vi "Begin.vi"(8 "error in":errorcluster) -> (0 "error out":errorcluster)   [LabVIEW 2016]
doc: "Called before other user functions, this VI is expected to open initial I/O refnums, load in file data, and do all program initialization. Notice that the <B>error out</B> terminal is simply used for data flow. Wiring it to other structures or subVIs ensures that this VI runs first."
uses:
  <vilib>/Rock Robotics/WPI/Camera/WPI_CameraImageSize.ctl
  <vilib>/Rock Robotics/WPI/DriverStation/WPI_DriverStationRobotMode2.ctl
  <vilib>/Rock Robotics/WPI/Joystick/WPI_JoystickDeviceEnum.ctl
  <vilib>/Rock Robotics/WPI/ThirdParty/CanMotor/TalonSRX/WPI_CANTalonSRX_BrakeOverride.ctl
  <vilib>/Rock Robotics/WPI/Solenoid/WPI_SolenoidChannel.ctl
  <vilib>/Rock Robotics/SystemInterfaces/DIO/FPGA_DIOChannel.ctl
  <vilib>/Rock Robotics/SystemInterfaces/DIO/FPGA_DIOPWMChannel.ctl
  <vilib>/Rock Robotics/WPI/ThirdParty/CanMotor/TalonSRX/WPI_CANTalonSRX_StatusFrame.ctl
  <vilib>/Rock Robotics/SystemInterfaces/AI/FPGA_AIChannel.ctl
  <vilib>/Rock Robotics/SystemInterfaces/DIO/FPGA_DIORelayChannel.ctl
  <vilib>/Rock Robotics/SystemInterfaces/spilib/spi_bus.ctl
  Robot Global Data.vi
  <vilib>/Rock Robotics/WPI/Utilities/WPI_GetSetVariantRefNum.vi
  <vilib>/Rock Robotics/WPI/Solenoid/WPI_SolenoidOpenSingle.vi
  <vilib>/Rock Robotics/WPI/MotorControl/WPI_MotorControlOpen VictorSP.vi
  <vilib>/Rock Robotics/WPI/Counter/WPI_CounterDigitalInputToDigitalSource.vi
  navX.Library.v2/navX Library v2/IO/Open/Z900_navX_Open_SPI.vi
  <vilib>/Rock Robotics/WPI/ThirdParty/CanMotor/TalonSRX/WPI_CANTalonSRX_APIControlMode.ctl
  <vilib>/Rock Robotics/WPI/Camera/WPI_CameraWhite Balance Values.ctl
  <vilib>/Rock Robotics/WPI/Camera/WPI_CameraExposure Values.ctl
  <vilib>/Rock Robotics/WPI/Ultrasonic/WPI_SonarSRF04DigitalOpen.vi
  <vilib>/Rock Robotics/WPI/Ultrasonic/WPI_SonarSRF04DigitalRefNum Registry Set.vi
  navX-MXP Library/navX-MXP IMU.lvlib
  navX-MXP Library/COMMON/TypeDefs/Value TypeDefs/navX Interface Protocol.ctl
  navX-MXP Library/COMMON/TypeDefs/Value TypeDefs/navX Update Rate.ctl
  <vilib>/Rock Robotics/WPI/AnalogOutput/WPI_AnalogOutputChannel.ctl
  <vilib>/Rock Robotics/WPI/Camera/WPI_CameraFrameRate.ctl
  navX.Library.v2/navX Library v2/navX Library v2.lvlib
  <vilib>/Rock Robotics/WPI/MotorControl/WPI_MotorControlOpen SD540.vi
panel:
  in  "Image Size":T1=enum."320x240"
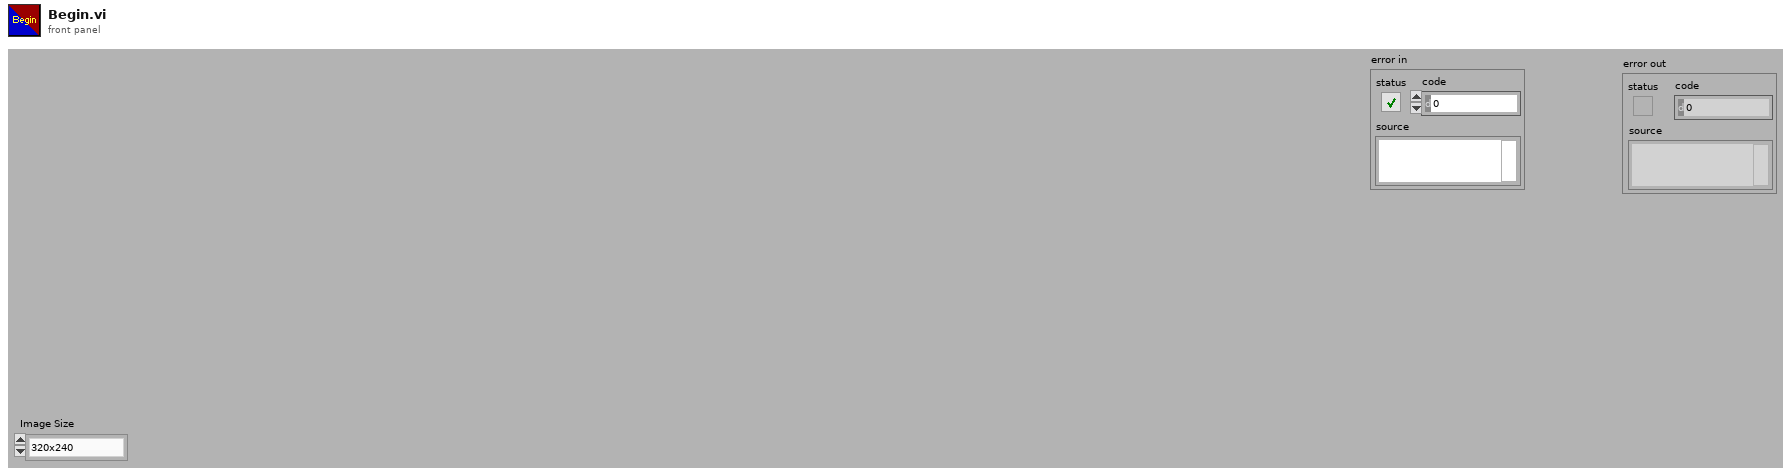
[diagram p1: front panel]
types:
  T1 = typedef "WPI_CameraImageSize.ctl" = enum16{"640x480", "320x240", "160x120", "Custom"}
  T2 = typedef "FPGA_DIORelayChannel.ctl" = enum8{"Relay 0", "Relay 1", "Relay 2", "Relay 3", "Invalid"}
  T3 = typedef "FPGA_DIOPWMChannel.ctl" = enum8{"PWM 0", "PWM 1", "PWM 2", "PWM 3", "PWM 4", "PWM 5", "PWM 6", "PWM 7", "PWM 8", "PWM 9", "PWM MXP 0", "PWM MXP 1", "PWM MXP 2", "PWM MXP 3", "PWM MXP 4", "PWM MXP 5", "PWM MXP 6", "PWM MXP 7", "PWM MXP 8", "PWM MXP 9", "Invalid"}
  T4 = typedef "WPI_SolenoidChannel.ctl" = enum8{"Solenoid 0", "Solenoid 1", "Solenoid 2", "Solenoid 3", "Solenoid 4", "Solenoid 5", "Solenoid 6", "Solenoid 7", "Invalid"}
  T5 = typedef "FPGA_AIChannel.ctl" = enum8{"AI 0", "AI 1", "AI 2", "AI 3", "AI MXP 0", "AI MXP 1", "AI MXP 2", "AI MXP 3", "Invalid"}
  T6 = typedef "WPI_CANTalonSRX_StatusFrame.ctl" = enum16{"General Status Frame", "Feedback Status Frame", "Quadrature Status Frame", "Analog Temp Vbat Status Frame", "Pulse Width Status Frame"}
  T7 = typedef "WPI_CANTalonSRX_BrakeOverride.ctl" = enum8{"No Override", "Override to Coast", "Override to Brake"}
  T8 = typedef "FPGA_DIOChannel.ctl" = enum8{"DIO 0", "DIO 1", "DIO 2", "DIO 3", "DIO 4", "DIO 5", "DIO 6", "DIO 7", "DIO 8", "DIO 9", "DIO MXP 0", "DIO MXP 1", "DIO MXP 2", "DIO MXP 3", "DIO MXP 4", "DIO MXP 5", "DIO MXP 6", "DIO MXP 7", "DIO MXP 8", "DIO MXP 9", "DIO MXP 10", "DIO MXP 11", "DIO MXP 12", "DIO MXP 13", "DIO MXP 14", "DIO MXP 15", "SPI Port CS1", "SPI Port CS2", "SPI Port CS3", "SPI Port MISO", "SPI Port MOSI", "Invalid"}
  T9 = typedef "WPI_JoystickDeviceEnum.ctl" = enum16{"USB 0", "USB 1", "USB 2", "USB 3", "USB 4", "USB 5"}
  T10 = typedef "WPI_DriverStationRobotMode2.ctl" = enum16{"Autonomous Disabled", "Autonomous Enabled", "Teleop Disabled", "Teleop Enabled", "Disconnected", "Finish", "Test Disabled", "Test Enabled", "Emergency Stopped"}
  T11 = typedef "navX-MXP IMU.lvlib/navX Update Rate.ctl" = u8
  T12 = typedef "navX-MXP IMU.lvlib/navX Interface Protocol.ctl" = enum16{"SPI", "I2C"}
  T13 = typedef "spi_bus.ctl" = enum16{"SPI On-Board, CS0", "SPI On-Board, CS1", "SPI On-Board, CS2", "SPI On-Board, CS3", "SPI MXP", "Invalid"}
  T14 = typedef "navX-MXP IMU.lvlib/navX Device TypeDef.ctl" = cluster{"navX Interface Protocol":T12, "navX Interface Protocol TypeDefs":cluster{"SPIDevRef":T15, "I2CDevRef":T16}, "navX System Information":cluster{"Board Information":T18, "Status":T19, "Offsets":T23}, "navX Common Information":cluster{"Update Rate (4Hz-60Hz)":T11, "refnum name":string, "error":errorcluster}}
  T15 = typedef "WPI_SPIDevRef.ctl" = cluster{"DevStatus":errorcluster, "Handle":i32, "SPI Bus":T13}
  T16 = typedef "WPI_I2CDevRef.ctl" = cluster{"DevStatus":errorcluster, "Device Address":u8, "Handle":i32, "I2C Bus":T17}
  T17 = typedef "i2c_bus.ctl" = enum16{"I2C On-Board", "I2C MXP", "Invalid"}
  T18 = typedef "navX-MXP IMU.lvlib/navX Board Information.ctl" = cluster{"WhoAmI (50 | 0x32)":u8, "Board Revision":u8, "Firmware Major Version":u8, "Firmware Minor Version":u8}
  T19 = typedef "navX-MXP IMU.lvlib/navX Status Data.ctl" = cluster{"Update Rate Hz":u8, "Accelerometer Full-Scale Range":u8, "Gyro Full-Scale Range":u16, "NAVX_OP_STATUS":T20, "NAVX_CAL_STATUS":T21, "NAVX_SELFTEST_STATUS":u8, "NAVX_SENSOR_STATUS":T22}
  T20 = typedef "navX-MXP IMU.lvlib/navX NAVX_OP_STATUS.ctl" = u8
  T21 = typedef "navX-MXP IMU.lvlib/navX NAVX_CAL_STATUS.ctl" = u8
  T22 = typedef "navX-MXP IMU.lvlib/navX NAVX_SENSOR_STATUS.ctl" = cluster{"MOVING":bool, "YAW_STABLE":bool, "MAG_DISTURBANCE":bool, "ALTITUDE_VALID":bool, "SEALEVEL_PRESS_SET":bool, "FUSED_HEADING_VALID":bool}
  T23 = typedef "navX-MXP IMU.lvlib/navX Offsets Data.ctl" = cluster{"Yaw":dbl, "Quat W":dbl, "Quat X":dbl, "Quat Y":dbl, "Quat Z":dbl}
  T24 = typedef "navX Library v2.lvlib/Z900_navX_DeviceTypeDef.ctl" = cluster{"Interface":cluster{"Protocol":T25, "Update Rate (4Hz-100Hz)":u8, "navX Open TypeDef":variant}, "Notify Packet":refnum<notifier>, "Loop VI Refnum":refnum<vi>, "Ready to Close Occurrence Refnum":refnum<k4>}
  T25 = typedef "navX Library v2.lvlib/Z900_navX_ProtocolTypeDef.ctl" = enum16{"SERIAL", "I2C", "SPI"}
  T26 = typedef "WPI_CameraExposure Values.ctl" = enum16{"Auto", "Flicker-free 50 Hz", "Flicker-free 60 Hz", "Hold current", "Custom"}
  T27 = typedef "WPI_CameraWhite Balance Values.ctl" = enum16{"Auto", "Fixed indoor", "Fixed outdoor 1", "Fixed outdoor 2", "Fixed fluorescent 1", "Fixed fluorescent 2", "Hold current", "Custom"}
  T28 = typedef "WPI_CameraFrameRate.ctl" = u32
  T29 = typedef "WPI_CameraDevRef.ctl" = cluster{"Camera Address":string, "CameraStatus":errorcluster}
  T30 = typedef "WPI_DigitalInputDevRef.ctl" = cluster{"DevStatus":errorcluster, "DIO Channel":T8}
  T31 = typedef "FPGA_CounterEncoderSourceConvertionLVSourceType.ctl" = cluster{"DevStatus":errorcluster, "AnalogTriggerMode?":bool, "DigitalMode":cluster{"DIO Channel":T32}, "AnalogTriggerMode":cluster{"AnalogTriggerIndex":T33, "OutputType":T34}}
  T32 = typedef "FPGA_DIODigitalSourceChannel.ctl" = enum8{"DIO 0", "DIO 1", "DIO 2", "DIO 3", "DIO 4", "DIO 5", "DIO 6", "DIO 7", "DIO 8", "DIO 9", "DIO MXP 0", "DIO MXP 1", "DIO MXP 2", "DIO MXP 3", "DIO MXP 4", "DIO MXP 5", "DIO MXP 6", "DIO MXP 7", "DIO MXP 8", "DIO MXP 9", "DIO MXP 10", "DIO MXP 11", "DIO MXP 12", "DIO MXP 13", "DIO MXP 14", "DIO MXP 15", "Disabled"}
  T33 = typedef "FPGA_AnalogTriggerIndex.ctl" = enum8{"Trig 0", "Trig 1", "Trig 2", "Trig 3", "Trig 4", "Trig 5", "Trig 6", "Trig 7", "Invalid"}
  T34 = typedef "FPGA_AnalogTriggerOutType.ctl" = enum16{"InWindow", "TriggerState", "Rising", "Falling"}
  T35 = typedef "WPI_SolenoidDevRef.ctl" = cluster{"DevStatus":errorcluster, "Pneumatics Control Module":u8, "Forward Solenoid Channel":T4, "Reverse Solenoid Channel":T4}
  T36 = typedef "WPI_EncoderDevRef.ctl" = cluster{"DevStatus":errorcluster, "EncoderIndex":T37, "CounterIndex":T38, "DistancePerCount":dbl, "Decoding Type":T39}
  T37 = typedef "FPGA_EncoderIdx.ctl" = enum8{"Enc 0", "Enc 1", "Enc 2", "Enc 3", "Enc 4", "Enc 5", "Enc 6", "Enc 7", "Invalid"}
  T38 = typedef "FPGA_CounterCtrSystemIndex.ctl" = enum8{"Ctr 0", "Ctr 1", "Ctr 2", "Ctr 3", "Ctr 4", "Ctr 5", "Ctr 6", "Ctr 7", "Invalid"}
  T39 = typedef "WPI_EncoderType.ctl" = enum16{"1x", "2x", "4x"}
  T40 = typedef "WPI_UltrasonicDeviceRef.ctl" = cluster{"DevStatus":errorcluster, "Ping Channel":T8, "Echo Channel":T8, "CntIndex":T38}
  T41 = typedef "WPI_CompressorDevRef.ctl" = cluster{"DevStatus":errorcluster, "Pneumatics Control Module":u8}
  T42 = typedef "WPI_JoystickDevRef.ctl" = cluster{"Device":T9}
  T43 = typedef "WPI_MotorControlDeviceRef.ctl" = cluster{"DeviceStatus":errorcluster, "Type":T44, "PWM":cluster{"PWM Channel":T3, "DeadBand":T45}, "CAN":cluster{"Device Number":u8, "SetOutput VI Ref":variant, "GetOutput VI Ref":variant, "Enable VI Ref":variant, "Disable VI Ref":variant, "Data":variant}, "Invert":bool}
  T44 = typedef "WPI_MotorControlType.ctl" = enum16{"PWM", "CAN"}
  T45 = typedef "WPI_PWMDeadband.ctl" = cluster{"Name":string, "maxPositivePwm":i32, "minPositivePwm":i32, "centerPwm":i32, "maxNegativePwm":i32, "minNegativePwm":i32, "angularRange":u16}
  T46 = typedef "WPI_AnalogChannelDevRef.ctl" = cluster{"DevStatus":errorcluster, "Analog Channel":T5}
  T47 = typedef "WPI_CANTalonSRX_APIControlMode.ctl" = enum8{"Percent VBus", "Speed", "Position", "Slave", "Unchanged / Invalid", "Voltage Compensation", "Current", "Motion Profile", "Motion Magic"}
  T48 = typedef "WPI_ServoDeviceRef.ctl" = cluster{"DeviceStatus":errorcluster, "PWM Channel":T3, "DeadBand":T45}
  T49 = typedef "WPI_AnalogOutputChannel.ctl" = enum8{"AO MXP 0", "AO MXP 1", "Invalid"}
  T50 = typedef "WPI_AOChannelDevRef.ctl" = cluster{"DevStatus":errorcluster, "AO Channel":T49}
  T51 = typedef "WPI_DigitalOutputDevRef.ctl" = cluster{"DIO Channel":T8, "DevStatus":errorcluster}
  T52 = typedef "WPI_RelayDevRef.ctl" = cluster{"DevStatus":errorcluster, "Relay Channel":T2, "Relay Direction":T53}
  T53 = typedef "WPI_RelayDirection.ctl" = enum16{"Both directions", "Forward only", "Reverse only"}
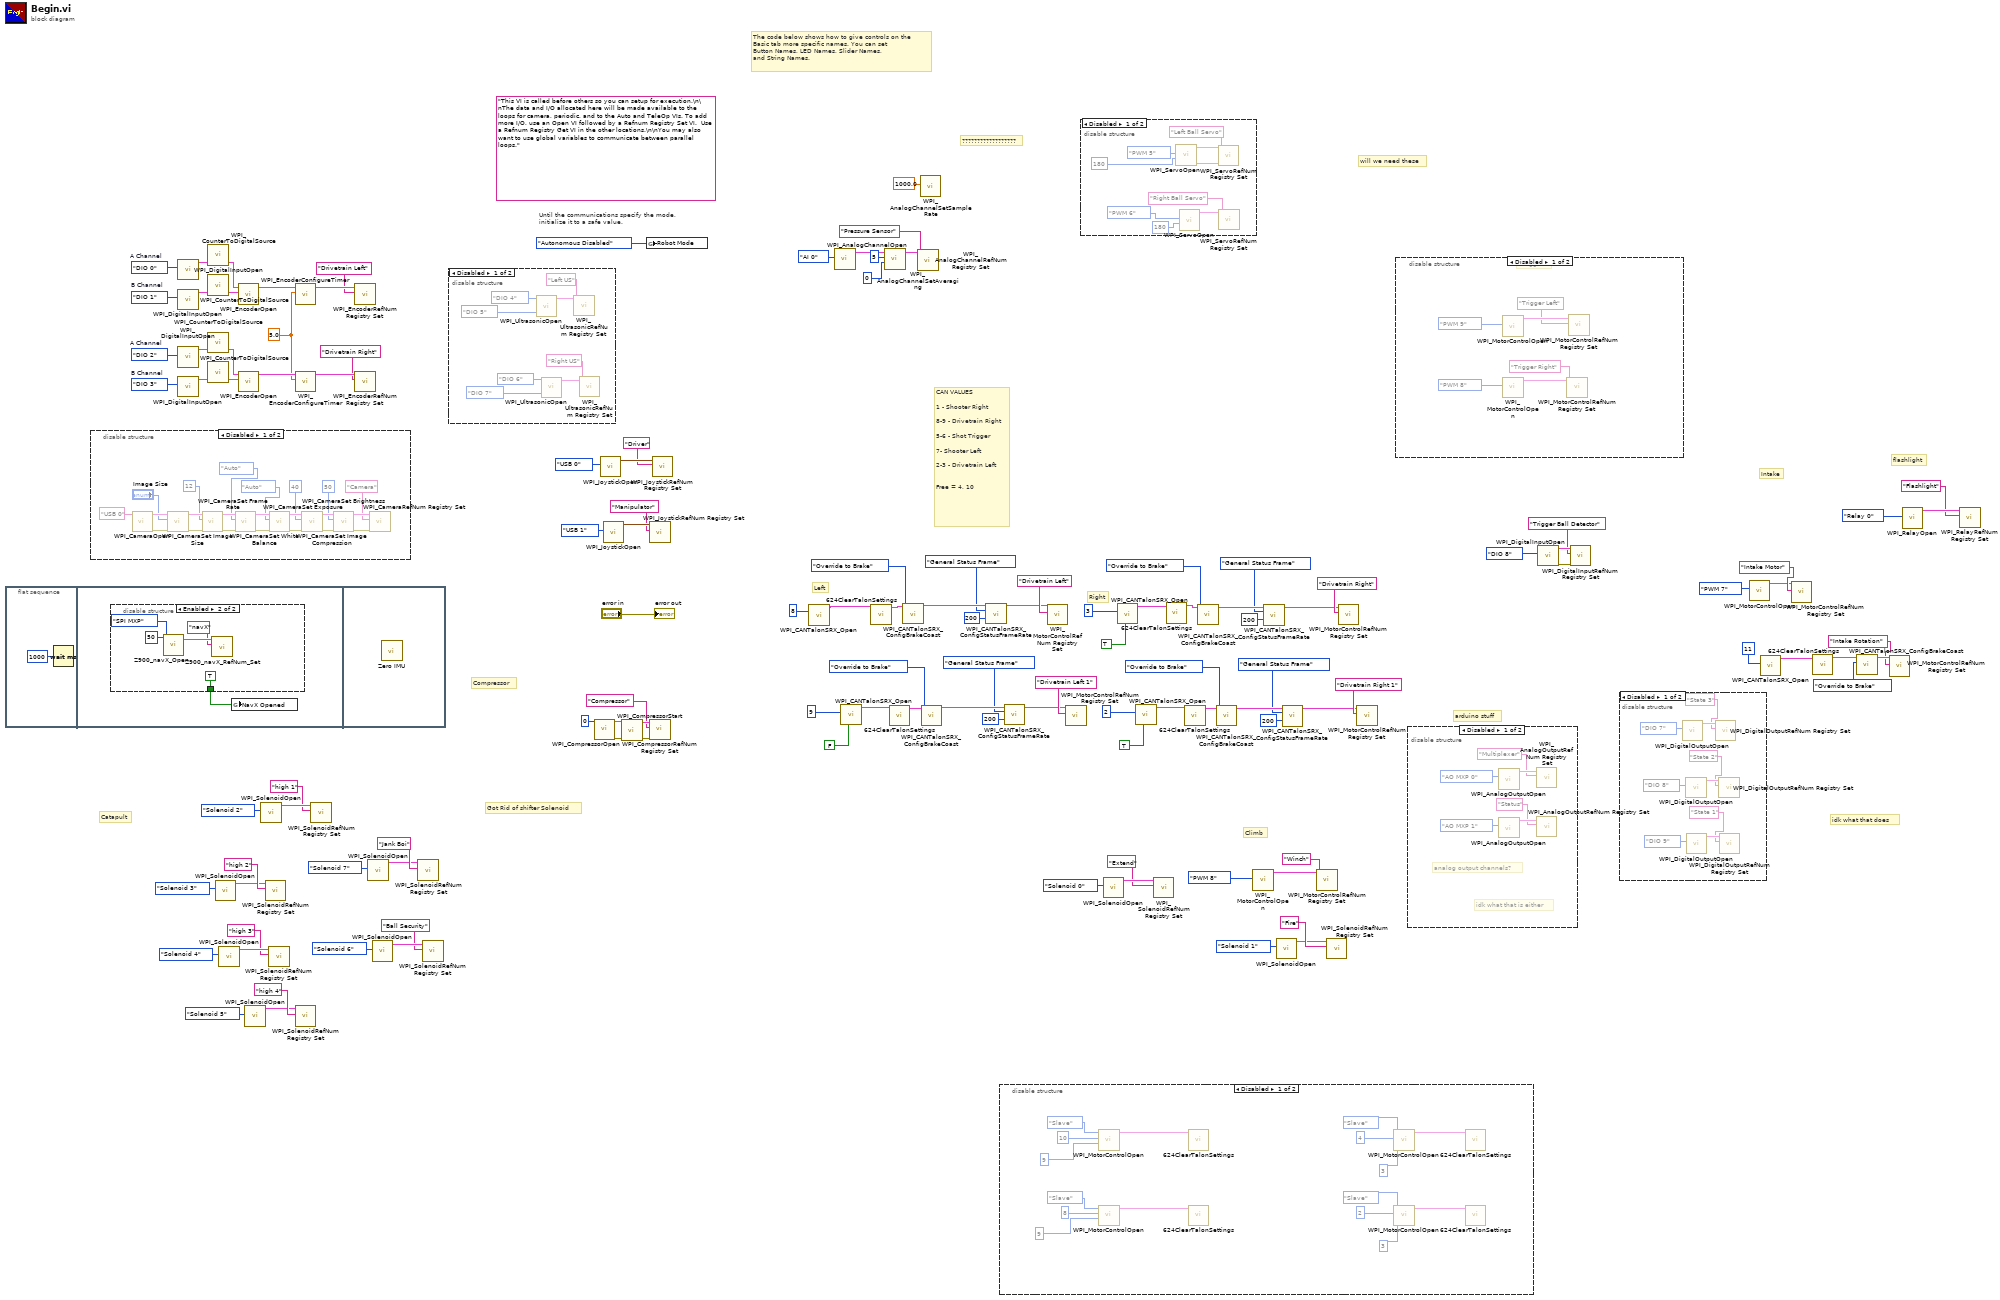
[diagram p0: block diagram]
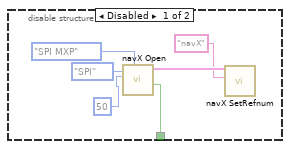
[diagram p9: hidden frame]
diagram:
  w66 = FPGA_DIOChannel."DIO 3"  # B Channel
  w69 = FPGA_DIOChannel."DIO 0"  # A Channel
  w72 = FPGA_DIOChannel."DIO 1"  # B Channel
  w77 = 5.0 ("Minimum Rate")
  w80 = FPGA_DIOChannel."DIO 2"  # A Channel
  (unwired) "This VI is called before others so you can setup for execution.\n\nThe data and I/O allocated here will be made available to the loops for camera, periodic, and to the Auto and TeleOp VIs. To add more I/O, use an Open VI followed by a Refnum Registry Set VI.  Use a Refnum Registry Get VI in the other locations.\n\nYou may also want to use global variables to communicate between parallel loops."
  # "flashlight"
  # "arduino stuff"
  # "Climb"
  # "will we need these"
  # "idk what that does"
  # "Got Rid of shifter Solenoid"
  # "Catapult"
  # "??????????????????"
  # "CAN VALUES\n\n1 - Shooter Right\n\n8-9 - Drivetrain Right\n\n5-6 - Shot Trigger\n\n7- Shooter Left\n\n2-3 - Drivetrain Left\n\n\nFree = 4, 10"
  # "Intake"
  # "Left"
  # "Right"
  # "Compressor"
  # "The code below shows how to give controls on the\nBasic tab more specific names. You can set\nButton Names, LED Names, Slider Names,\nand String Names."
  # "Until the communications specify the mode,\ninitialize it to a safe value."
  n1 = flat-sequence {
    frame #0 {
      n2 = Wait (ms)(milliseconds to wait=u32 1000) -> ()  [unwired: 1 out]
    }
    frame #1 {
      n3 = disable-structure shown="Enabled" {
        disable-tunnel: [w125 TRUE ("NavX Opened")] -> w124
        frame Disabled {
          n4 = call "navX Open.vi"("SPI Bus"=spi_bus."SPI MXP", "Update Rate (4Hz-60Hz)"=T11 50, "navX Interface Protocol"=navX_Interface_Protocol."SPI") -> ("Opened?"=w125:bool, "navX Device TypeDef"=w130:T14)  [unwired: 6 in, 1 out]
          n5 = call "navX SetRefnum.vi"("refnum name"="navX", "navX Device TypeDef"=w130) -> ()  [unwired: 8 in, 2 out]
        }
        frame Enabled {
          n6 = call-poly "Z900_navX_Open.vi"("SPI Bus"=spi_bus."SPI MXP", "Update Rate (4Hz-60Hz)"=u8 50) -> ("navX Device"=w135:T24)  [unwired: 8 in, 1 out]
          n7 = call "Z900_navX_RefNum_Set.vi"("refnum name"="navX", "navX Device"=w135) -> ()  [unwired: 8 in, 2 out]
        }
      }
      n8 = global write "Robot Global Data.vi" "NavX Opened"(w124) -> ()
    }
    frame #2 {
      n9 = call "Zero IMU.vi"() -> ()  [unwired: 12 in]
    }
  }
  n10 = disable-structure shown="Disabled" {
    frame Disabled {
      n11 = call <vilib>:"WPI_CameraOpen.vi"("Camera Address"="USB 0" ("format string")) -> ("error out"=w145:errorcluster, "CameraDevRef"=w144:T29)  [unwired: 1 in, 8 out]
      n12 = call <vilib>:"WPI_CameraSet Image Size.vi"("error in (no error)"=w145, "Image Size"="Image Size", "CameraDevRef"=w144) -> ("error out"=w147:errorcluster, "CameraDevRef Out"=w146:T29)  [unwired: 1 in, 6 out]
      n13 = call <vilib>:"WPI_CameraSet Frame Rate.vi"("error in (no error)"=w147, "Frame Rate (fps)"=T28 12, "CameraDevRef"=w146) -> ("error out"=w149:errorcluster, "CameraDevRef Out"=w148:T29)  [unwired: 7 out]
      n14 = call <vilib>:"WPI_CameraSet White Balance.vi"("error in (no error)"=w149, "White Balance"=WPI_CameraWhite_Balance_Values."Auto", "CameraDevRef"=w148) -> ("error out"=w151:errorcluster, "CameraDevRef Out"=w150:T29)  [unwired: 1 in, 6 out]
      n15 = call <vilib>:"WPI_CameraSet Exposure.vi"("error in (no error)"=w151, "Exposure"=WPI_CameraExposure_Values."Auto", "CameraDevRef"=w150) -> ("error out"=w153:errorcluster, "CameraDevRef Out"=w152:T29)  [unwired: 1 in, 6 out]
      n16 = call <vilib>:"WPI_CameraSet Image Compression.vi"("error in (no error)"=w153, "Compression"=40, "CameraDevRef"=w152) -> ("error out"=w155:errorcluster, "CameraDevRef Out"=w154:T29)  [unwired: 7 out]
      n17 = call <vilib>:"WPI_CameraSet Brightness.vi"("error in (no error)"=w155, "Brightness"=50, "CameraDevRef"=w154) -> ("error out"=w157:errorcluster, "CameraDevRef Out"=w156:T29)  [unwired: 7 out]
      n18 = call <vilib>:"WPI_CameraRefNum Registry Set.vi"("error in (no error)"=w157, "refnum name"="Camera", "CameraDevRef"=w156) -> ()  [unwired: 1 in, 8 out]
    }
    frame Enabled {
    }
  }
  n19 = call <vilib>:"WPI_DigitalInputOpen.vi"("DIO Channel"=w69) -> ("DigitalInputDevRef"=w70:T30)  [unwired: 1 in, 9 out]
  n20 = call <vilib>:"WPI_DigitalInputOpen.vi"("DIO Channel"=w72) -> ("DigitalInputDevRef"=w73:T30)  [unwired: 1 in, 9 out]
  n21 = call <vilib>:"WPI_DigitalInputOpen.vi"("DIO Channel"=w80) -> ("DigitalInputDevRef"=w81:T30)  [unwired: 1 in, 9 out]
  n22 = call <vilib>:"WPI_DigitalInputOpen.vi"("DIO Channel"=w66) -> ("DigitalInputDevRef"=w78:T30)  [unwired: 1 in, 9 out]
  n23 = call-poly <vilib>:"WPI_CounterToDigitalSource.vi"("DigitalInputDevRef"=w70) -> ("Digital Source"=w71:T31)  [unwired: 6 out]
  n24 = call-poly <vilib>:"WPI_CounterToDigitalSource.vi"("DigitalInputDevRef"=w73) -> ("Digital Source"=w74:T31)  [unwired: 6 out]
  n25 = call-poly <vilib>:"WPI_CounterToDigitalSource.vi"("DigitalInputDevRef"=w81) -> ("Digital Source"=w82:T31)  [unwired: 6 out]
  n26 = call-poly <vilib>:"WPI_CounterToDigitalSource.vi"("DigitalInputDevRef"=w78) -> ("Digital Source"=w79:T31)  [unwired: 6 out]
  n27 = call-poly <vilib>:"WPI_SolenoidOpen.vi"("Solenoid Channel"=WPI_SolenoidChannel."Solenoid 3") -> ("SolenoidDevRef"=w26:T35)  [unwired: 9 in, 1 out]
  n28 = call-poly <vilib>:"WPI_SolenoidOpen.vi"("Solenoid Channel"=WPI_SolenoidChannel."Solenoid 4") -> ("SolenoidDevRef"=w23:T35)  [unwired: 9 in, 1 out]
  n29 = call <vilib>:"WPI_EncoderOpen.vi"("BSource"=w74, "ASource"=w71) -> ("EncoderDevRef"=w75:T36)  [unwired: 6 in, 3 out]
  n30 = call <vilib>:"WPI_EncoderOpen.vi"("BSource"=w79, "ASource"=w82) -> ("EncoderDevRef"=w83:T36)  [unwired: 6 in, 3 out]
  n31 = call-poly <vilib>:"WPI_SolenoidOpen.vi"("Solenoid Channel"=WPI_SolenoidChannel."Solenoid 5") -> ("SolenoidDevRef"=w20:T35)  [unwired: 9 in, 1 out]
  n32 = call-poly <vilib>:"WPI_SolenoidOpen.vi"("Solenoid Channel"=WPI_SolenoidChannel."Solenoid 2") -> ("SolenoidDevRef"=w29:T35)  [unwired: 9 in, 1 out]
  n33 = call <vilib>:"WPI_SolenoidRefNum Registry Set.vi"("refnum name"="high 2", "SolenoidDevRef"=w26) -> ()  [unwired: 8 in, 2 out]
  n34 = call <vilib>:"WPI_SolenoidRefNum Registry Set.vi"("refnum name"="high 3", "SolenoidDevRef"=w23) -> ()  [unwired: 8 in, 2 out]
  n35 = call <vilib>:"WPI_EncoderConfigureTimer.vi"("Minimum Rate"=w77, "EncoderDevRef"=w75) -> ("EncoderDevRef"=w76:T36)  [unwired: 8 in, 1 out]
  n36 = call <vilib>:"WPI_EncoderConfigureTimer.vi"("Minimum Rate"=w77, "EncoderDevRef"=w83) -> ("EncoderDevRef"=w84:T36)  [unwired: 8 in, 1 out]
  n37 = call <vilib>:"WPI_SolenoidRefNum Registry Set.vi"("refnum name"="high 4", "SolenoidDevRef"=w20) -> ()  [unwired: 8 in, 2 out]
  n38 = call <vilib>:"WPI_SolenoidRefNum Registry Set.vi"("refnum name"="high 1", "SolenoidDevRef"=w29) -> ()  [unwired: 8 in, 2 out]
  n39 = call <vilib>:"WPI_EncoderRefNum Registry Set.vi"("refnum name"="Drivetrain Left", "EncoderDevRef"=w76) -> ()  [unwired: 8 in, 2 out]
  n40 = call <vilib>:"WPI_EncoderRefNum Registry Set.vi"("refnum name"="Drivetrain Right", "EncoderDevRef"=w84) -> ()  [unwired: 8 in, 2 out]
  n41 = call-poly <vilib>:"WPI_SolenoidOpen.vi"("Solenoid Channel"=WPI_SolenoidChannel."Solenoid 7") -> ("SolenoidDevRef"=w15:T35)  [unwired: 9 in, 1 out]
  n42 = call-poly <vilib>:"WPI_SolenoidOpen.vi"("Solenoid Channel"=WPI_SolenoidChannel."Solenoid 6") -> ("SolenoidDevRef"=w18:T35)  [unwired: 9 in, 1 out]
  n43 = call <vilib>:"WPI_SolenoidRefNum Registry Set.vi"("refnum name"="Jank Boi", "SolenoidDevRef"=w15) -> ()  [unwired: 8 in, 2 out]
  n44 = call <vilib>:"WPI_SolenoidRefNum Registry Set.vi"("refnum name"="Ball Security", "SolenoidDevRef"=w18) -> ()  [unwired: 8 in, 2 out]
  n45 = disable-structure shown="Disabled" {
    frame Disabled {
      n46 = call-poly <vilib>:"WPI_UltrasonicOpen.vi"("Echo DIO Channel"=FPGA_DIOChannel."DIO 5", "Ping DIO Channel"=FPGA_DIOChannel."DIO 4") -> ("SonarSRF04DevRef"=w165:T40)  [unwired: 8 in, 1 out]
      n47 = call-poly <vilib>:"WPI_UltrasonicOpen.vi"("Echo DIO Channel"=FPGA_DIOChannel."DIO 7", "Ping DIO Channel"=FPGA_DIOChannel."DIO 6") -> ("SonarSRF04DevRef"=w158:T40)  [unwired: 8 in, 1 out]
      n48 = call-poly <vilib>:"WPI_UltrasonicRefNum Registry Set.vi"("refnum name"="Left US", "SonarSRF04DevRef"=w165) -> ()  [unwired: 8 in, 2 out]
      n49 = call-poly <vilib>:"WPI_UltrasonicRefNum Registry Set.vi"("refnum name"="Right US", "SonarSRF04DevRef"=w158) -> ()  [unwired: 8 in, 2 out]
    }
    frame Enabled {
    }
  }
  n50 = call <vilib>:"WPI_CompressorOpen.vi"("Pneumatics Control Module (0)"=0) -> ("CompressorDevRef"=w117:T41, "error out"=w114:errorcluster)  [unwired: 13 in]
  n51 = call <vilib>:"WPI_JoystickOpen.vi"("JoystickDevice"=WPI_JoystickDeviceEnum."USB 0") -> ("JoystickDevRef"=w121:T42)  [unwired: 10 in]
  n52 = call <vilib>:"WPI_JoystickOpen.vi"("JoystickDevice"=WPI_JoystickDeviceEnum."USB 1") -> ("JoystickDevRef"=w104:T42)  [unwired: 10 in]
  n53 = call <vilib>:"WPI_CompressorStart.vi"("error in (no error)"=w114, "CompressorDevRef"=w117) -> ("error out"=w113:errorcluster, "CompressorDevRef"=w116:T41)  [unwired: 8 in]
  n54 = global write "Robot Global Data.vi" "Robot Mode"(WPI_DriverStationRobotMode2."Autonomous Disabled" ("Robot Mode")) -> ()
  n55 = call <vilib>:"WPI_JoystickRefNum Registry Set.vi"("refnum name"="Manipulator", "JoystickDevRef"=w104) -> ()  [unwired: 8 in, 2 out]
  n56 = call <vilib>:"WPI_CompressorRefNum Registry Set.vi"("error in (no error)"=w113, "refnum name"="Compressor", "CompressorDevRef"=w116) -> ()  [unwired: 7 in, 2 out]
  n57 = call <vilib>:"WPI_JoystickRefNum Registry Set.vi"("refnum name"="Driver", "JoystickDevRef"=w121) -> ()  [unwired: 8 in, 2 out]
  n58 = call <vilib>:"WPI_CANTalonSRX_Open.vi"("Device Number"=8) -> ("CAN Talon SRX Ref"=w5:T43)  [unwired: 9 in, 1 out]
  n59 = call <vilib>:"WPI_AnalogChannelOpen.vi"("Analog Channel"=FPGA_AIChannel."AI 0") -> ("AIDeviceRef"=w38:T46)  [unwired: 9 in, 1 out]
  n60 = call <vilib>:"WPI_CANTalonSRX_Open.vi"("Invert"=FALSE, "Device Number"=9) -> ("CAN Talon SRX Ref"=w107:T43)  [unwired: 8 in, 1 out]
  n61 = call "624ClearTalonSettings.vi"("CAN Talon SRX Ref Out"=w5) -> ("CAN Talon SRX Ref Out 2"=w50:T43)  [unwired: 10 in]
  n62 = call <vilib>:"WPI_AnalogChannelSetAveraging.vi"("OversampleBits"=u8 0, "AverageBits"=u8 5, "AIDeviceRef"=w38) -> ("AIDeviceRef"=w37:T46)  [unwired: 7 in, 1 out]
  n63 = call "624ClearTalonSettings.vi"("CAN Talon SRX Ref Out"=w107) -> ("CAN Talon SRX Ref Out 2"=w108:T43)  [unwired: 10 in]
  n64 = call <vilib>:"WPI_CANTalonSRX_ConfigBrakeCoast.vi"("Brake / Coast Mode"=WPI_CANTalonSRX_BrakeOverride."Override to Brake", "CAN Talon SRX Ref"=w50) -> ("CAN Talon SRX Ref"=w45:T43)  [unwired: 8 in, 1 out]
  n65 = call <vilib>:"WPI_AnalogChannelRefNum Registry Set.vi"("refnum name"="Pressure Sensor", "AIDeviceRef"=w37) -> ()  [unwired: 8 in, 2 out]
  n66 = call <vilib>:"WPI_AnalogChannelSetSampleRate.vi"("Samples Per Second (per channel)"=1000.0) -> ()  [unwired: 10 in, 1 out]
  n67 = call <vilib>:"WPI_CANTalonSRX_ConfigBrakeCoast.vi"("Brake / Coast Mode"=WPI_CANTalonSRX_BrakeOverride."Override to Brake", "CAN Talon SRX Ref"=w108) -> ("CAN Talon SRX Ref"=w63:T43)  [unwired: 8 in, 1 out]
  n68 = call <vilib>:"WPI_CANTalonSRX_ConfigStatusFrameRate.vi"("CAN Talon SRX Ref"=w45, "Talon SRX Status Frame"=WPI_CANTalonSRX_StatusFrame."General Status Frame", "Frame Rate Ms"=u32 200) -> ("CAN Talon SRX Ref"=w44:T43)  [unwired: 12 in]
  n69 = disable-structure shown="Disabled" {
    frame Disabled {
      n70 = call-poly <vilib>:"WPI_MotorControlOpen.vi"("Eliminate Deadband"=u8 9 ("Master Device Number"), "PWM Channel"=u8 10 ("Device Number"), 11:WPI_CANTalonSRX_APIControlMode."Slave" ("Control Mode")) -> ("MotorControlDeviceRef"=w173:T43)  [unwired: 7 in, 1 out]
      n71 = call-poly <vilib>:"WPI_MotorControlOpen.vi"("Eliminate Deadband"=u8 9 ("Master Device Number"), "PWM Channel"=u8 8 ("Device Number"), 11:WPI_CANTalonSRX_APIControlMode."Slave" ("Control Mode")) -> ("MotorControlDeviceRef"=w174:T43)  [unwired: 7 in, 1 out]
      n72 = call "624ClearTalonSettings.vi"("CAN Talon SRX Ref Out"=w173) -> ()  [unwired: 10 in, 1 out]
      n73 = call "624ClearTalonSettings.vi"("CAN Talon SRX Ref Out"=w174) -> ()  [unwired: 10 in, 1 out]
      n74 = call-poly <vilib>:"WPI_MotorControlOpen.vi"("Eliminate Deadband"=u8 3 ("Master Device Number"), "PWM Channel"=u8 4 ("Device Number"), 11:WPI_CANTalonSRX_APIControlMode."Slave" ("Control Mode")) -> ("MotorControlDeviceRef"=w166:T43)  [unwired: 7 in, 1 out]
      n75 = call-poly <vilib>:"WPI_MotorControlOpen.vi"("Eliminate Deadband"=u8 3 ("Master Device Number"), "PWM Channel"=u8 2 ("Device Number"), 11:WPI_CANTalonSRX_APIControlMode."Slave" ("Control Mode")) -> ("MotorControlDeviceRef"=w181:T43)  [unwired: 7 in, 1 out]
      n76 = call "624ClearTalonSettings.vi"("CAN Talon SRX Ref Out"=w166) -> ()  [unwired: 10 in, 1 out]
      n77 = call "624ClearTalonSettings.vi"("CAN Talon SRX Ref Out"=w181) -> ()  [unwired: 10 in, 1 out]
    }
    frame Enabled {
    }
  }
  n78 = call <vilib>:"WPI_CANTalonSRX_ConfigStatusFrameRate.vi"("CAN Talon SRX Ref"=w63, "Talon SRX Status Frame"=WPI_CANTalonSRX_StatusFrame."General Status Frame", "Frame Rate Ms"=u32 200) -> ("CAN Talon SRX Ref"=w62:T43)  [unwired: 12 in]
  n79 = call <vilib>:"WPI_MotorControlRefNum Registry Set.vi"("refnum name"="Drivetrain Left", "MotorControlDevRef"=w44) -> ()  [unwired: 8 in, 2 out]
  n80 = call <vilib>:"WPI_MotorControlRefNum Registry Set.vi"("refnum name"="Drivetrain Left 1", "MotorControlDevRef"=w62) -> ()  [unwired: 8 in, 2 out]
  n81 = disable-structure shown="Disabled" {
    frame Disabled {
      n82 = call <vilib>:"WPI_ServoOpen.vi"("Angular Range"=u16 180, "PWM Channel"=FPGA_DIOPWMChannel."PWM 5") -> ("error out"=w188:errorcluster, "ServoDeviceRef"=w187:T48)  [unwired: 8 in]
      n83 = call <vilib>:"WPI_ServoOpen.vi"("Angular Range"=u16 180, "PWM Channel"=FPGA_DIOPWMChannel."PWM 6") -> ("ServoDeviceRef"=w186:T48)  [unwired: 8 in, 1 out]
      n84 = call <vilib>:"WPI_ServoRefNum Registry Set.vi"("error in (no error)"=w188, "refnum name"="Left Ball Servo", "ServoDeviceRef"=w187) -> ()  [unwired: 7 in, 2 out]
      n85 = call <vilib>:"WPI_ServoRefNum Registry Set.vi"("refnum name"="Right Ball Servo", "ServoDeviceRef"=w186) -> ()  [unwired: 8 in, 2 out]
    }
    frame Enabled {
    }
  }
  n86 = call-poly <vilib>:"WPI_SolenoidOpen.vi"("Solenoid Channel"=WPI_SolenoidChannel."Solenoid 0") -> ("SolenoidDevRef"=w93:T35)  [unwired: 9 in, 1 out]
  n87 = call <vilib>:"WPI_CANTalonSRX_Open.vi"("Invert"=TRUE, "Device Number"=3) -> ("CAN Talon SRX Ref"=w52:T43)  [unwired: 8 in, 1 out]
  n88 = call <vilib>:"WPI_CANTalonSRX_Open.vi"("Invert"=TRUE, "Device Number"=2) -> ("CAN Talon SRX Ref"=w110:T43)  [unwired: 8 in, 1 out]
  n89 = call <vilib>:"WPI_SolenoidRefNum Registry Set.vi"("refnum name"="Extend", "SolenoidDevRef"=w93) -> ()  [unwired: 8 in, 2 out]
  n90 = call "624ClearTalonSettings.vi"("CAN Talon SRX Ref Out"=w52) -> ("CAN Talon SRX Ref Out 2"=w51:T43)  [unwired: 10 in]
  n91 = call "624ClearTalonSettings.vi"("CAN Talon SRX Ref Out"=w110) -> ("CAN Talon SRX Ref Out 2"=w109:T43)  [unwired: 10 in]
  n92 = call <vilib>:"WPI_CANTalonSRX_ConfigBrakeCoast.vi"("Brake / Coast Mode"=WPI_CANTalonSRX_BrakeOverride."Override to Brake", "CAN Talon SRX Ref"=w51) -> ("CAN Talon SRX Ref"=w47:T43)  [unwired: 8 in, 1 out]
  n93 = call <vilib>:"WPI_CANTalonSRX_ConfigBrakeCoast.vi"("Brake / Coast Mode"=WPI_CANTalonSRX_BrakeOverride."Override to Brake", "CAN Talon SRX Ref"=w109) -> ("CAN Talon SRX Ref"=w65:T43)  [unwired: 8 in, 1 out]
  n94 = call-poly <vilib>:"WPI_MotorControlOpen.vi"("PWM Channel"=FPGA_DIOPWMChannel."PWM 8") -> ("MotorControlDeviceRef"=w11:T43)  [unwired: 9 in, 1 out]
  n95 = call <vilib>:"WPI_CANTalonSRX_ConfigStatusFrameRate.vi"("CAN Talon SRX Ref"=w47, "Talon SRX Status Frame"=WPI_CANTalonSRX_StatusFrame."General Status Frame", "Frame Rate Ms"=u32 200) -> ("CAN Talon SRX Ref"=w46:T43)  [unwired: 12 in]
  n96 = call-poly <vilib>:"WPI_SolenoidOpen.vi"("Solenoid Channel"=WPI_SolenoidChannel."Solenoid 1") -> ("SolenoidDevRef"=w59:T35)  [unwired: 9 in, 1 out]
  n97 = call <vilib>:"WPI_CANTalonSRX_ConfigStatusFrameRate.vi"("CAN Talon SRX Ref"=w65, "Talon SRX Status Frame"=WPI_CANTalonSRX_StatusFrame."General Status Frame", "Frame Rate Ms"=u32 200) -> ("CAN Talon SRX Ref"=w64:T43)  [unwired: 12 in]
  n98 = call <vilib>:"WPI_MotorControlRefNum Registry Set.vi"("refnum name"="Winch", "MotorControlDevRef"=w11) -> ()  [unwired: 8 in, 2 out]
  n99 = call <vilib>:"WPI_SolenoidRefNum Registry Set.vi"("refnum name"="Fire", "SolenoidDevRef"=w59) -> ()  [unwired: 8 in, 2 out]
  n100 = call <vilib>:"WPI_MotorControlRefNum Registry Set.vi"("refnum name"="Drivetrain Right", "MotorControlDevRef"=w46) -> ()  [unwired: 8 in, 2 out]
  n101 = call <vilib>:"WPI_MotorControlRefNum Registry Set.vi"("refnum name"="Drivetrain Right 1", "MotorControlDevRef"=w64) -> ()  [unwired: 8 in, 2 out]
  n102 = disable-structure shown="Disabled" {
    frame Disabled {
      # "\"Trigger\""
      n103 = call-poly <vilib>:"WPI_MotorControlOpen.vi"("PWM Channel"=FPGA_DIOPWMChannel."PWM 9") -> ("MotorControlDeviceRef"=w194:T43)  [unwired: 9 in, 1 out]
      n104 = call-poly <vilib>:"WPI_MotorControlOpen.vi"("PWM Channel"=FPGA_DIOPWMChannel."PWM 8") -> ("MotorControlDeviceRef"=w193:T43)  [unwired: 9 in, 1 out]
      n105 = call <vilib>:"WPI_MotorControlRefNum Registry Set.vi"("refnum name"="Trigger Right", "MotorControlDevRef"=w193) -> ()  [unwired: 8 in, 2 out]
      n106 = call <vilib>:"WPI_MotorControlRefNum Registry Set.vi"("refnum name"="Trigger Left", "MotorControlDevRef"=w194) -> ()  [unwired: 8 in, 2 out]
    }
    frame Enabled {
    }
  }
  n107 = disable-structure shown="Disabled" {
    frame Disabled {
      # "analog output channels?"
      # "idk what that is either"
      n108 = call <vilib>:"WPI_AnalogOutputOpen.vi"("AO Channel"=WPI_AnalogOutputChannel."AO MXP 0") -> ("AODeviceRef"=w199:T50)  [unwired: 9 in, 1 out]
      n109 = call <vilib>:"WPI_AnalogOutputOpen.vi"("AO Channel"=WPI_AnalogOutputChannel."AO MXP 1") -> ("AODeviceRef"=w202:T50)  [unwired: 9 in, 1 out]
      n110 = call <vilib>:"WPI_AnalogOutputRefNum Registry Set.vi"("refnum name"="Multiplexer", "AODeviceRef"=w199) -> ()  [unwired: 8 in, 2 out]
      n111 = call <vilib>:"WPI_AnalogOutputRefNum Registry Set.vi"("refnum name"="Status", "AODeviceRef"=w202) -> ()  [unwired: 8 in, 2 out]
    }
    frame Enabled {
    }
  }
  n112 = call <vilib>:"WPI_DigitalInputOpen.vi"("DIO Channel"=FPGA_DIOChannel."DIO 8") -> ("error out"=w89:errorcluster, "DigitalInputDevRef"=w88:T30)  [unwired: 9 in]
  n113 = call <vilib>:"WPI_DigitalInputRefNum Registry Set.vi"("error in (no error)"=w89, "refnum name"="Trigger Ball Detector", "DigitalInputDevRef"=w88) -> ()  [unwired: 7 in, 2 out]
  n114 = disable-structure shown="Disabled" {
    frame Disabled {
      n115 = call <vilib>:"WPI_DigitalOutputOpen.vi"("DIO Channel"=FPGA_DIOChannel."DIO 7") -> ("DigitalOutputDevRef"=w205:T51)  [unwired: 9 in, 1 out]
      n116 = call <vilib>:"WPI_DigitalOutputOpen.vi"("DIO Channel"=FPGA_DIOChannel."DIO 8") -> ("DigitalOutputDevRef"=w208:T51)  [unwired: 9 in, 1 out]
      n117 = call <vilib>:"WPI_DigitalOutputOpen.vi"("DIO Channel"=FPGA_DIOChannel."DIO 9") -> ("DigitalOutputDevRef"=w211:T51)  [unwired: 9 in, 1 out]
      n118 = call <vilib>:"WPI_DigitalOutputRefNum Registry Set.vi"("refnum name"="State 3", "DigitalOutputDevRef"=w205) -> ()  [unwired: 8 in, 2 out]
      n119 = call <vilib>:"WPI_DigitalOutputRefNum Registry Set.vi"("refnum name"="State 2", "DigitalOutputDevRef"=w208) -> ()  [unwired: 8 in, 2 out]
      n120 = call <vilib>:"WPI_DigitalOutputRefNum Registry Set.vi"("refnum name"="State 1", "DigitalOutputDevRef"=w211) -> ()  [unwired: 8 in, 2 out]
    }
    frame Enabled {
    }
  }
  n121 = call-poly <vilib>:"WPI_MotorControlOpen.vi"("PWM Channel"=FPGA_DIOPWMChannel."PWM 7") -> ("MotorControlDeviceRef"=w85:T43)  [unwired: 9 in, 1 out]
  n122 = call <vilib>:"WPI_CANTalonSRX_Open.vi"("Device Number"=u8 11) -> ("CAN Talon SRX Ref"=w97:T43)  [unwired: 9 in, 1 out]
  n123 = call <vilib>:"WPI_MotorControlRefNum Registry Set.vi"("refnum name"="Intake Motor", "MotorControlDevRef"=w85) -> ()  [unwired: 8 in, 2 out]
  n124 = call "624ClearTalonSettings.vi"("CAN Talon SRX Ref Out"=w97) -> ("CAN Talon SRX Ref Out 2"=w98:T43)  [unwired: 10 in]
  n125 = call <vilib>:"WPI_CANTalonSRX_ConfigBrakeCoast.vi"("Brake / Coast Mode"=WPI_CANTalonSRX_BrakeOverride."Override to Brake", "CAN Talon SRX Ref"=w98) -> ("CAN Talon SRX Ref"=w99:T43)  [unwired: 8 in, 1 out]
  n126 = call <vilib>:"WPI_MotorControlRefNum Registry Set.vi"("refnum name"="Intake Rotation", "MotorControlDevRef"=w99) -> ()  [unwired: 8 in, 2 out]
  n127 = call <vilib>:"WPI_RelayOpen.vi"("Relay Channel"=FPGA_DIORelayChannel."Relay 0") -> ("RelayDevRef"=w9:T52)  [unwired: 9 in, 1 out]
  n128 = call <vilib>:"WPI_RelayRefNum Registry Set.vi"("refnum name"="Flashlight", "RelayDevRef"=w9) -> ()  [unwired: 8 in, 2 out]
  "error out" <- "error in"
